vi "Sandstorm.vi"(10 "Normal Game":T2, 11 "Turn Number in":i32) -> (3 "Sandstorm":T1)   [LabVIEW 2018]
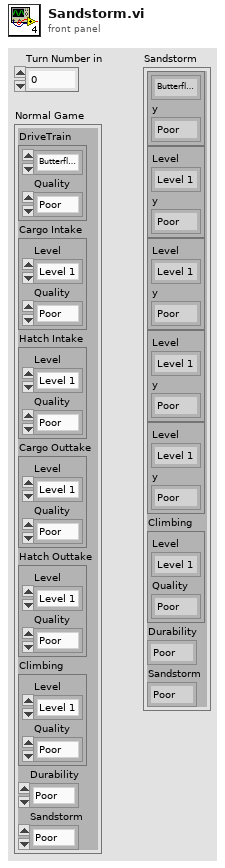
[diagram p1: front panel]
types:
  T1 = cluster{cluster{enum16{"Butterfly Tank/H-Drive", "Butterfly-Tank/Tank", "Tread", "Strafe", "Swerve", "Tank Traction"}, "y":enum16{"Poor", "Good", "Excellent"}}, cluster{"Level":enum16{"Level 1", "Level 2", "Level 3"}, "y":enum16{"Poor", "Good", "Excellent"}}, cluster{"Level":enum16{"Level 1", "Level 2", "Level 3"}, "y":enum16{"Poor", "Good", "Excellent"}}, cluster{"Level":enum16{"Level 1", "Level 2", "Level 3"}, "y":enum16{"Poor", "Good", "Excellent"}}, cluster{"Level":enum16{"Level 1", "Level 2", "Level 3"}, "y":enum16{"Poor", "Good", "Excellent"}}, "Climbing":cluster{"Level":enum16{"Level 1", "Level 2", "Level 3"}, "Quality":enum16{"Poor", "Good", "Excellent"}}, "Durability":enum16{"Poor", "Good", "Excellent"}, "Sandstorm":enum16{"Poor", "Good", "Excellent"}}
  T2 = cluster{"DriveTrain":cluster{enum16{"Butterfly Tank/H-Drive", "Butterfly-Tank/Tank", "Tread", "Strafe", "Swerve", "Tank Traction"}, "Quality":enum16{"Poor", "Good", "Excellent"}}, "Cargo Intake":cluster{"Level":enum16{"Level 1", "Level 2", "Level 3"}, "Quality":enum16{"Poor", "Good", "Excellent"}}, "Hatch Intake":cluster{"Level":enum16{"Level 1", "Level 2", "Level 3"}, "Quality":enum16{"Poor", "Good", "Excellent"}}, "Cargo Outtake":cluster{"Level":enum16{"Level 1", "Level 2", "Level 3"}, "Quality":enum16{"Poor", "Good", "Excellent"}}, "Hatch Outtake":cluster{"Level":enum16{"Level 1", "Level 2", "Level 3"}, "Quality":enum16{"Poor", "Good", "Excellent"}}, "Climbing":cluster{"Level":enum16{"Level 1", "Level 2", "Level 3"}, "Quality":enum16{"Poor", "Good", "Excellent"}}, "Durability":enum16{"Poor", "Good", "Excellent"}, "Sandstorm":enum16{"Poor", "Good", "Excellent"}}
  T3 = cluster{enum16{"Butterfly Tank/H-Drive", "Butterfly-Tank/Tank", "Tread", "Strafe", "Swerve", "Tank Traction"}, "Quality":enum16{"Poor", "Good", "Excellent"}}
  T4 = cluster{"Level":enum16{"Level 1", "Level 2", "Level 3"}, "Quality":enum16{"Poor", "Good", "Excellent"}}
  T5 = enum16{"Butterfly Tank/H-Drive", "Butterfly-Tank/Tank", "Tread", "Strafe", "Swerve", "Tank Traction"}
  T6 = cluster{enum16{"Butterfly Tank/H-Drive", "Butterfly-Tank/Tank", "Tread", "Strafe", "Swerve", "Tank Traction"}, "y":enum16{"Poor", "Good", "Excellent"}}
  T7 = cluster{"Level":enum16{"Level 1", "Level 2", "Level 3"}, "y":enum16{"Poor", "Good", "Excellent"}}
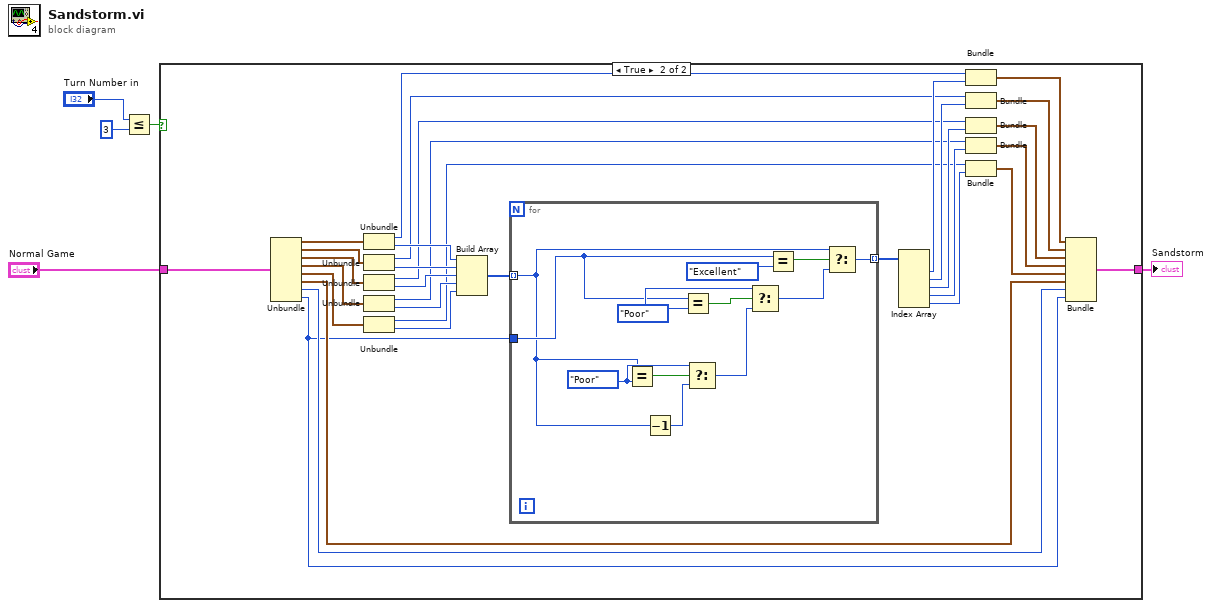
[diagram p0: block diagram]
diagram:
  n1 = Less Or Equal?(x="Turn Number in", y=3) -> (x <= y?=w2:bool)
  n2 = case shown="True" w2 {
    tunnel: "Normal Game" -> [w6 w38]
    tunnel: [w6 w7] -> w5
    frame False {
    }
    frame True {
      n3 = Unbundle(w38) -> ("DriveTrain"=w37:T3, "Cargo Intake"=w36:T4, "Hatch Intake"=w35:T4, "Cargo Outtake"=w34:T4, "Hatch Outtake"=w33:T4, "Climbing"=w10:T4, "Durability"=w9:enum16{"Poor", "Good", "Excellent"}, "Sandstorm"=w8:enum16{"Poor", "Good", "Excellent"})
      n4 = Unbundle(w37) -> (w16:T5, "Quality"=w32:enum16{"Poor", "Good", "Excellent"})
      n5 = Unbundle(w36) -> ("Level"=w17:enum16{"Level 1", "Level 2", "Level 3"}, "Quality"=w31:enum16{"Poor", "Good", "Excellent"})
      n6 = Unbundle(w35) -> ("Level"=w18:enum16{"Level 1", "Level 2", "Level 3"}, "Quality"=w30:enum16{"Poor", "Good", "Excellent"})
      n7 = Unbundle(w34) -> ("Level"=w19:enum16{"Level 1", "Level 2", "Level 3"}, "Quality"=w29:enum16{"Poor", "Good", "Excellent"})
      n8 = Unbundle(w33) -> ("Level"=w20:enum16{"Level 1", "Level 2", "Level 3"}, "Quality"=w28:enum16{"Poor", "Good", "Excellent"})
      n9 = Build Array(w32, w31, w30, w29, w28) -> (w27:enum16{"Poor", "Good", "Excellent"}[])
      n10 = for {
        tunnel: w27 -> [w40] mode=indexing
        tunnel: w8 -> [w41]
        tunnel: [w39] -> w26 mode=indexing
        w44 = enum16{"Poor", "Good", "Excellent"}."Poor"
        w43 = enum16{"Poor", "Good", "Excellent"}."Poor" ("y")
        n11 = Equal?(x=w40, y=w44) -> (x = y?=w47:bool)
        n12 = Decrement(x=w40) -> (x-1=w45:enum16{"Poor", "Good", "Excellent"})
        n13 = Equal?(x=w41, y=w43) -> (x = y?=w49:bool)
        n14 = Select(t=w44, s=w47, f=w45) -> (s? t:f=w46:enum16{"Poor", "Good", "Excellent"})
        n15 = Select(t=w43, s=w49, f=w46) -> (s? t:f=w48:enum16{"Poor", "Good", "Excellent"})
        n16 = Equal?(x=w41, y=enum16{"Poor", "Good", "Excellent"}."Excellent") -> (x = y?=w50:bool)
        n17 = Select(t=w40, s=w50, f=w48) -> (s? t:f=w39:enum16{"Poor", "Good", "Excellent"})
      }
      n18 = Index Array(array=w26) -> (element #1=w25:enum16{"Poor", "Good", "Excellent"}, element #2=w21:enum16{"Poor", "Good", "Excellent"}, element #3=w22:enum16{"Poor", "Good", "Excellent"}, element #4=w23:enum16{"Poor", "Good", "Excellent"}, element #5=w24:enum16{"Poor", "Good", "Excellent"})  [unwired: 5 in]
      n19 = Bundle(w16, "y"=w25) -> (w15:T6)  [unwired: 1 in]
      n20 = Bundle("Level"=w17, "y"=w21) -> (w14:T7)  [unwired: 1 in]
      n21 = Bundle("Level"=w18, "y"=w22) -> (w13:T7)  [unwired: 1 in]
      n22 = Bundle("Level"=w19, "y"=w23) -> (w12:T7)  [unwired: 1 in]
      n23 = Bundle("Level"=w20, "y"=w24) -> (w11:T7)  [unwired: 1 in]
      n24 = Bundle(w15, w14, w13, w12, w11, "Climbing"=w10, "Durability"=w9, "Sandstorm"=w8) -> (w7:T1)  [unwired: 1 in]
    }
  }
  "Sandstorm" <- w5
